vi "NI VeriStand - Save Configuration File.vi"(8 "Error in":errorcluster, 11 "Runtime Configuration Ref in":refnum<k24>) -> (0 "Error out":errorcluster, 2 "Success":bool, 3 "Runtime Configuration Ref out":refnum<k24>)   [LabVIEW 2025, in "NI_VS RuntimeConfigurationFile ScriptingAPI.lvlib"]
uses:
  NI_VS RuntimeConfigurationFile ScriptingAPI.lvlib
  NationalInstruments.VeriStand.SystemDefinitionAPI
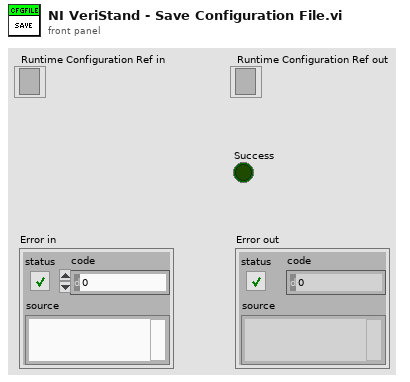
[diagram p1: front panel]
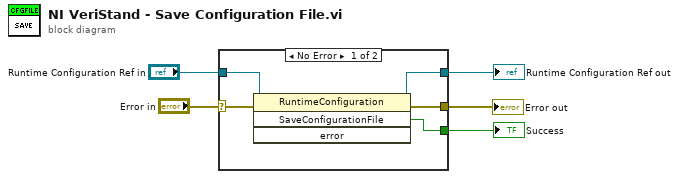
[diagram p0: block diagram]
diagram:
  n1 = case shown="No Error" "Error in" {
    selector: "Error in" -> [w9 _]
    tunnel: "Runtime Configuration Ref in" -> [w8 w11]
    tunnel: [w7 w11] -> w2
    tunnel: [w6 _] -> w1
    tunnel: [w10 _] -> w5
    frame No Error {
      n2 = invoke class="RuntimeConfiguration" method="SaveConfigurationFile"(reference=w8, error in=w9) -> (reference out=w7:refnum<k24>, error out=w10:errorcluster, "SaveConfigurationFile"=w6:bool)  [unwired: 2 in, 1 out]
    }
    frame Error {
    }
  }
  "Runtime Configuration Ref out" <- w2
  "Success" <- w1
  "Error out" <- w5
